vi "Helicopter - 3DView.vi"() -> ()   [LabVIEW 2013]
doc: "Sample numeric display item."
uses:
  <vilib>/NI Veristand/Display Template Support/Display Template Support.llb/cluster_Screen Item Settings.ctl
  <vilib>/NI Veristand/Display Template Support/Display Template Support.llb/cluster_Graph Scale Settings.ctl
  <vilib>/NI Veristand/Display Template Support/Display Template Support.llb/cluster_Graph Plot Settings.ctl
  NationalInstruments.VeriStand.SystemStorage
  <vilib>/NI Veristand/Display Template Support/Display Template Support.llb/enum_Display Template Handler Minimal To Widget Msg.ctl
  <vilib>/NI Veristand/Display Template Support/Display Template Support.llb/enum_Display Template Handler Minimal To Workspace.ctl
  <vilib>/Utility/sysdir.llb/System Directory Type.ctl
  Data.ctl
  <vilib>/NI Veristand/Execution/Workspace/NI_VS Workspace ExecutionAPI.lvlib
panel:
  in  "NIVS.System Definition Root":refnum<k24>
  in  "NIVS.Gateway IP Address":string
  out "Helicoptor Model":refnum<vi>(3d-picture)
  in  "Item.Data":T1
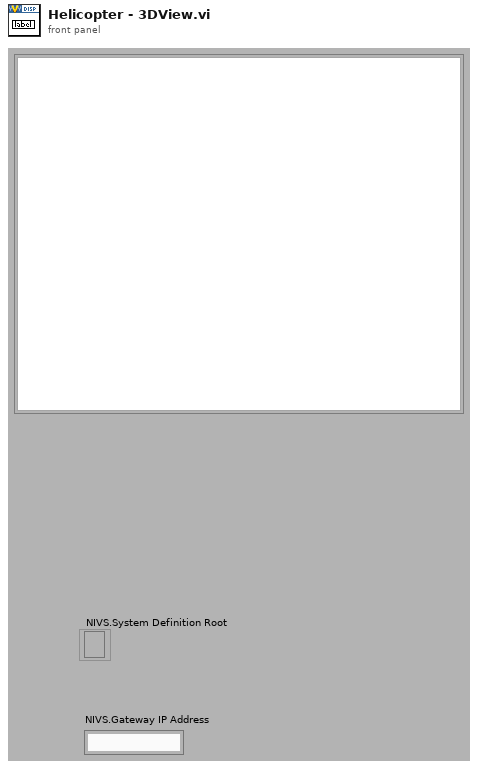
[diagram p1: front panel]
types:
  T1 = typedef "cluster_Screen Item Settings.ctl" = cluster{"Template VI":string, "Position X":i32, "Position Y":i32, "Custom":string, "Show Title Bar":bool, "ID":i32, "Always On Top":bool, "Allow Resize":bool, "Allow Minimize":bool, "Allow Close":bool, "Size to Screen":bool, "Screen.ID":i32, "State":enum16{"Normal", "New"}, "Title":string, "Window Bounds":cluster{"[0]":i16, "[1]":i16, "[2]":i16, "[3]":i16}, "Channel Ref":u64, "Unit":string, "Default Units?":bool, "Flash Limit?":bool, "Color 1":u32, "Color 2":u32, "Color 3":u32, "Color 4":u32, "Bck Color":u32, "Fore Color":u32, "Limit 1":dbl, "Limit 2":dbl, "Limit 3":dbl, "Limit 4":dbl, "Limit Mode 1":i32, "Limit Mode 2":i32, "Limit Mode 3":i32, "Limit Mode 4":i32, "Scale Precision":i32, "Scale Min":dbl, "Scale Max":dbl, "Format":i32, "Precision":i32, "Background Type":i32, "IDs":i32[], "Units":string[], "Labels":string[], "Scale Factor":dbl, "Scale Offset":dbl, "YScale Index":u32[], "XScale":T2, "YScales":T2[], "Plots":T3[], "Update Period":dbl, "History Length":dbl, "My.Ref":refnum<vi>, "Is Control?":bool, "Channel Paths":string[], "Custom Data":variant}
  T2 = typedef "cluster_Graph Scale Settings.ctl" = cluster{"Format":u8, "Precision":u8, "Fit":u8, "Label":string, "Use Default Label":bool, "Label Visible":bool, "Min":dbl, "Max":dbl}
  T3 = typedef "cluster_Graph Plot Settings.ctl" = cluster{"Bar Style":u8, "Fill To":i16, "Fill/PtColor":u32, "Line Style":u8, "Line Width":u8, "Color":u32, "Interp":u8, "Point Style":u8}
  T4 = typedef "Data.ctl" = cluster{"Elevation":string[], "Travel":string[], "Pitch":string[], "3D Model Path":path, "Elevation Flat Path":string, "Travel Flat Path":string, "Pitch Flat Path":string}
  T5 = typedef "System Directory Type.ctl" = i32
  T6 = typedef "enum_Display Template Handler Minimal To Workspace.ctl" = cluster{"Operation":enum16{"SetCustomData", "DeleteItem"}, "Data":variant}
  T7 = typedef "enum_Display Template Handler Minimal To Widget Msg.ctl" = enum16{"Stop", "LaunchConfigDialog"}
  T8 = typedef "NI_VS Workspace ExecutionAPI.lvlib/WorkspaceAPI.ctl" = refnum<k24>
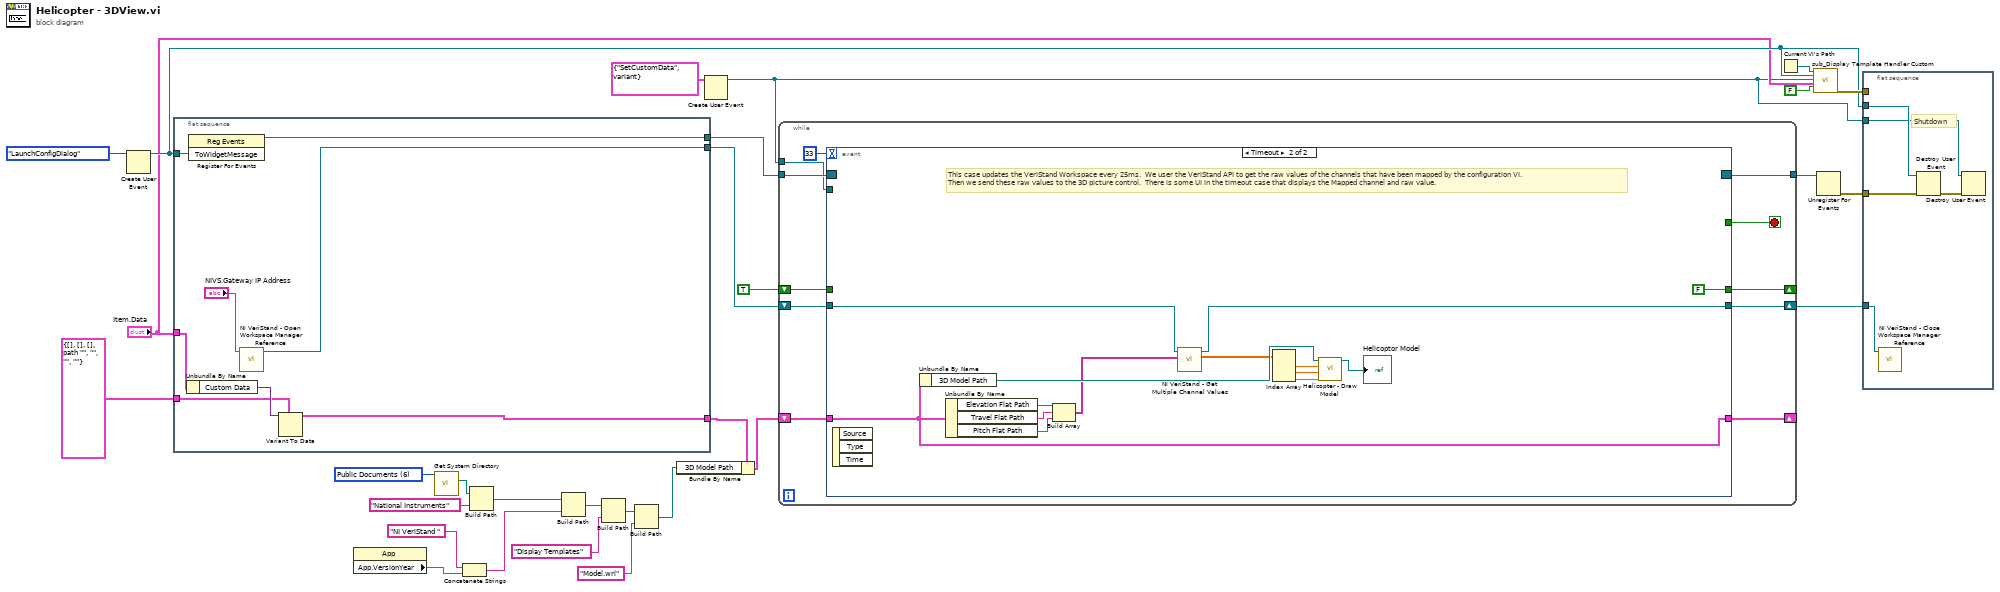
[diagram p0: block diagram]
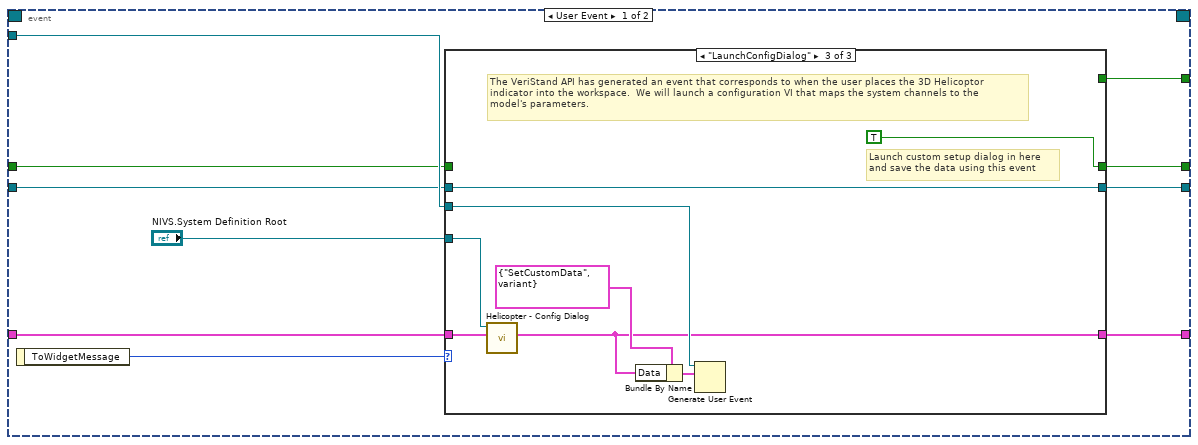
[diagram p2: hidden frame]
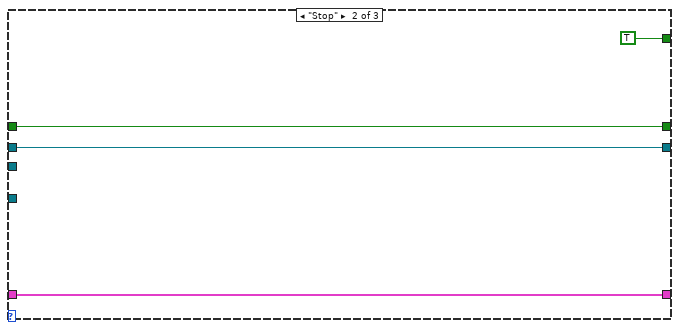
[diagram p4: hidden frame]
diagram:
  w8 = T5 6 items=["User Home", "User Desktop", "User Documents", "User Application Data", "User Preferences", "User Temporary", "Public Documents", "Public Application Data", "Public Preferences", "System Core Libraries", "System Installed Libraries", "Application Files", "Boot Volume Root"] ("system directory type")
  n1 = Create User Event(user event datatype=enum_Display_Template_Handler_Minimal_To_Widget_Msg."LaunchConfigDialog" ("ToWidgetMessage")) -> (user event=w24:refnum<user-event>)  [unwired: 1 in, 1 out]
  n2 = flat-sequence {
    tunnel: [w37] -> w27
    tunnel: w24 -> [w36]
    tunnel: "Item.Data" -> [w35]
    tunnel: [w31] -> w17
    tunnel: T4 {"Elevation"=[], "Travel"=[], "Pitch"=[], "3D Model Path"=path "", "Elevation Flat Path"="", "Travel Flat Path"="", "Pitch Flat Path"=""} ("Data") -> [w33]
    tunnel: [w32] -> w14
    frame #0 {
      n3 = Unbundle By Name(w35) -> ("Custom Data"=w34:variant)
      n4 = register-events(w36) -> (reference out=w37:refnum<event-registration>)  [unwired: 2 in, 1 out]
      n5 = call <vilib>:"NI VeriStand - Open Workspace Manager Reference.vi"("Gateway IP Address (\"\": localhost)"="NIVS.Gateway IP Address") -> ("WorkspaceManager"=w31:T8)  [unwired: 9 in, 1 out]
      n6 = Variant To Data(type=w33, Variant=w34) -> (data=w32:T4)  [unwired: 1 in, 1 out]
    }
  }
  n7 = property class="App"() -> ("App.VersionYear"=w2:string)  [unwired: 2 in, 2 out]
  n8 = call <vilib>:"Get System Directory.vi"("system directory type"=w8) -> ("system directory"=w7:path)  [unwired: 10 in]
  n9 = Concatenate Strings("NI VeriStand " ("name or relative path"), w2) -> (w1:string)
  n10 = Build Path(base path=w7, name or relative path="National Instruments") -> (appended path=w5:path)
  n11 = Build Path(base path=w5, name or relative path=w1) -> (appended path=w9:path)
  n12 = Build Path(base path=w9, name or relative path="Display Templates") -> (appended path=w11:path)
  n13 = Build Path(base path=w11, name or relative path="Model.wrl") -> (appended path=w4:path)
  n14 = Bundle By Name(cluster=w14, "3D Model Path"=w4) -> (w13:T4)
  n15 = Create User Event(user event datatype=T6 {"Operation"=enum."SetCustomData", "Data"=variant} ("Data")) -> (user event=w20:refnum<user-event>)  [unwired: 1 in, 1 out]
  n16 = while {
    tunnel: w27 -> [w48]
    tunnel: [w47] -> w26
    tunnel: w20 -> [w46]
    shift-right: [w39] -> _
    shift-left: w13 -> [w43]
    shift-right: [w42] -> w16
    shift-left: w17 -> [w44]
    shift-right: [w41] -> _
    shift-left: TRUE -> [w40]
    stop <- w38 stop-if-true
    n17 = event shown="[1] Timeout" {
      selector: w48 -> [_ _]
      dyn-events: [_ _] -> w47
      timeout: 33 -> [_ _]
      tunnel: [w57 _] -> w38
      tunnel: w46 -> [w56 _]
      tunnel: w44 -> [w51 w87]
      tunnel: w43 -> [w55 w85]
      tunnel: [w50 w86] -> w42
      tunnel: [w54 w85] -> w39
      tunnel: [w53 FALSE] -> w41
      tunnel: w40 -> [w52 _]
      event User Event {
        n18 = event-data() -> ("ToWidgetMessage"=w58:T7)  [unwired: 1 out]
        n19 = case shown="\"LaunchConfigDialog\"" w58 {
          tunnel: [_ TRUE _] -> w57
          tunnel: w56 -> [_ _ w73]
          tunnel: w55 -> [w61 w64 w72]
          tunnel: [w61 w64 w69] -> w54
          tunnel: [w60 w63 TRUE] -> w53
          tunnel: w52 -> [w60 w63 _]
          tunnel: w51 -> [w59 w62 w67]
          tunnel: [w59 w62 w67] -> w50
          tunnel: "NIVS.System Definition Root" -> [_ _ w66]
          frame Default {
          }
          frame "Stop" {
          }
          frame "LaunchConfigDialog" {
            # "The VeriStand API has generated an event that corresponds to when the user places the 3D Helicoptor \nindicator into the workspace.  We will launch a configuration VI that maps the system channels to the \nmodel's parameters."
            # "Launch custom setup dialog in here\nand save the data using this event"
            n20 = call "Helicopter - Config Dialog.vi"("In"=w72, "NIVS.System Definition Root"=w66) -> ("Out"=w69:T4)  [unwired: 8 in, 1 out]
            n21 = Bundle By Name(cluster=T6 {"Operation"=enum."SetCustomData", "Data"=variant} ("event data"), "Data"=w69) -> (w70:T6)
            n22 = Generate User Event(user event=w73, event data cluster=w70) -> ()  [unwired: 2 in, 2 out]
          }
        }
      }
      event Timeout {
        # "This case updates the VeriStand Workspace every 25ms.  We user the VeriStand API to get the raw values of the channels that have been mapped by the configuration VI.\nThen we send these raw values to the 3D picture control.  There is some UI in the timeout case that displays the Mapped channel and raw value."
        n23 = event-data() -> ()  [unwired: 4 out]
        n24 = Unbundle By Name(w85) -> ("3D Model Path"=w83:path)
        n25 = Unbundle By Name(w85) -> ("Elevation Flat Path"=w80:string, "Travel Flat Path"=w82:string, "Pitch Flat Path"=w81:string)
        n26 = Build Array(w80, w82, w81) -> (w79:string[])
        n27 = call <vilib>:"NI VeriStand - Get Multiple Channel Values.vi"("Channels"=w79, "WorkspaceManager in"=w87) -> ("Values"=w78:dbl[], "WorkspaceManager out"=w86:T8)  [unwired: 7 in, 1 out]
        n28 = Index Array(array=w78) -> (element #1=w76:dbl, element #2=w75:dbl, element #3=w74:dbl)  [unwired: 3 in]
        n29 = call "Helicopter - Draw Model.vi"("Pitch"=w74, "Travel"=w75, "Elevation"=w76, "Path to 3D model"=w83) -> ("Scene.New Object"=→"Helicoptor Model":refnum<vi>)  [unwired: 6 in, 1 out]
      }
    }
  }
  n30 = Current VI's Path() -> (path=w22:path)
  n31 = call <vilib>:"sub_Display Template Handler Custom.vi"("Parent.Path"=w22, "ToWidgetEvent"=w24, "ToWorkspace"=w20, "Item.Data"="Item.Data", "Resizable"=FALSE) -> ("error out"=w29:errorcluster)  [unwired: 14 in]
  n32 = Unregister For Events(event registration refnum=w26) -> (error out=w25:errorcluster)  [unwired: 1 in]
  n33 = flat-sequence {
    tunnel: w29 -> [_]
    tunnel: w25 -> [w91]
    tunnel: w24 -> [w92]
    tunnel: w20 -> [w89]
    tunnel: w16 -> [w88]
    frame #0 {
      # "Shutdown"
      n34 = call <vilib>:"NI VeriStand - Close Workspace Manager Reference.vi"("WorkspaceManager"=w88) -> ()  [unwired: 10 in, 1 out]
      n35 = Destroy User Event(user event=w92, error in=w91) -> (error out=w90:errorcluster)
      n36 = Destroy User Event(user event=w89, error in=w90) -> ()  [unwired: 1 out]
    }
  }
